vi "S4GUI.vi"() -> ()   [LabVIEW 2018] (continued)
                n1359 = call-dynamic "Read Interface.vi"("error in (no error)"=w3056, "Channel in"=w3057) -> ("error out"=w3047:errorcluster, "Interface.lvclass"=w3046:refnum<class "Interface.lvclass">, "Channel out"=w3059:refnum<class "Channel.lvclass">)  [unwired: 7 in]
                n1360 = call-dynamic "Get CCD_Config.vi"("error in (no error)"=w3047, "Interface in"=w3046) -> ("error out"=w3049:errorcluster, "output cluster"=w3050:T24, "Interface out"=w3045:refnum<class "Interface.lvclass">)  [unwired: 7 in]
                n1361 = Bundle By Name(cluster=w3050, "TRIGGER_MODE"=w3023) -> (w3048:T24)
                n1362 = call-dynamic "Set CCD_Config.vi"("error in (no error)"=w3049, "input cluster"=w3048, "Interface in"=w3045) -> ("error out"=w3051:errorcluster, "Interface out"=w3044:refnum<class "Interface.lvclass">)  [unwired: 7 in]
                n1363 = Flatten To String(anything=w3048, error in (no error)=w3051) -> (data string=w3053:string, error out=w3052:errorcluster)  [unwired: 2 in, 1 out]
                n1364 = call "Write flatted cluster.vi"("error in (no error)"=w3052, "flatted cluster"=w3053, "Interface in"=w3044) -> ("error out"=w3042:errorcluster, "Interface out"=w3043:refnum<class "Interface.lvclass">)  [unwired: 7 in]
                n1365 = call-dynamic "Write Interface.vi"("error in (no error)"=w3042, "Interface.lvclass"=w3043, "Channel in"=w3059) -> ("error out"=w3037:errorcluster, "Channel out"=w3036:refnum<class "Channel.lvclass">)  [unwired: 7 in]
                n1366 = call "Write section_name.vi"("error in (no error)"=w3037, "section_name"="CCD_ACS1", "Channel in"=w3036) -> ("error out"=w3038:errorcluster, "Channel out"=w3033:refnum<class "Channel.lvclass">)  [unwired: 7 in]
                n1367 = call-dynamic "save config.vi"("error in (no error)"=w3038, "file config"="lastsaved.cfg", "Channel in"=w3033) -> ("error out"=w3026:errorcluster, "Channel out"=w3027:refnum<class "Channel.lvclass">)  [unwired: 7 in]
                n1368 = call-dynamic "Read State Machine.vi"("error in (no error)"=w3026, "Device in"=w3027) -> ("error out"=w3041:errorcluster, "State Machine.lvclass"=w3031:refnum<class "State Machine.lvclass">, "Device out"=w3032:refnum<class "Channel.lvclass">)  [unwired: 7 in]
                n1369 = call-dynamic "Write State.vi"("error in (no error)"=w3041, "State"=60, "State Machine in"=w3031) -> ("error out"=w3040:errorcluster, "State Machine out"=w3030:refnum<class "State Machine.lvclass">)  [unwired: 7 in]
                n1370 = call-dynamic "Write State Machine.vi"("error in (no error)"=w3040, "State Machine.lvclass"=w3030, "Device in"=w3032) -> ("error out"=w3028:errorcluster, "Device out"=w3029:refnum<class "Channel.lvclass">)  [unwired: 7 in]
                n1371 = call-dynamic "Write Channel.vi"("error in (no error)"=w3028, "Channel.lvclass"=w3029, "Acquisition in"=w3058) -> ("error out"=w3055:errorcluster, "Acquisition out"=w3054:refnum<class "Acquisition.lvclass">)  [unwired: 7 in]
              }
            }
            n1372 = call-dynamic "Write AcquisitionA.vi"("error in (no error)"=w2860, "Acquisition.lvclass"=w2861, "S4ACS_GUI in"=w2862) -> ("error out"=w2868:errorcluster, "S4ACS_GUI out"=w2871:refnum<class "S4GUI.lvclass">)  [unwired: 7 in]
            n1373 = call "Write AcquisitionB.vi"("error in (no error)"=w2858, "Acquisition.lvclass"=w2859, "S4ACS_GUI in"=w2871) -> ("error out"=w2867:errorcluster, "S4ACS_GUI out"=w2870:refnum<class "S4GUI.lvclass">)  [unwired: 7 in]
            n1374 = call-dynamic "Write AcquisitionC.vi"("error in (no error)"=w2856, "Acquisition.lvclass"=w2857, "S4ACS_GUI in"=w2870) -> ("error out"=w2866:errorcluster, "S4ACS_GUI out"=w2869:refnum<class "S4GUI.lvclass">)  [unwired: 7 in]
            n1375 = call-dynamic "Write AcquisitionD.vi"("error in (no error)"=w2854, "Acquisition.lvclass"=w2855, "S4ACS_GUI in"=w2869) -> ("error out"=w2865:errorcluster, "S4ACS_GUI out"=w2864:refnum<class "S4GUI.lvclass">)  [unwired: 7 in]
            n1376 = Merge Errors(w2868, w2867, w2866, w2865) -> (w2863:errorcluster)
          }
        }
        n1377 = call-dynamic "Write sync.vi"("error in (no error)"=w2602, "sync"=w2628, "S4ACS_GUI in"=w2603) -> ("error out"=w2627:errorcluster, "S4ACS_GUI out"=w2604:refnum<class "S4GUI.lvclass">)  [unwired: 7 in]
        n1378 = property on="#Cycles Done" class="Slide (strict)"(error in=w2627, "DisabledEnum"=w2625) -> (error out=w2626:errorcluster)  [unwired: 1 in, 1 out]
        n1379 = property on="Cycles Done ch1" class="Slide (strict)"(error in=w2626, "DisabledEnum"=w2605) -> (error out=w2624:errorcluster)  [unwired: 1 in, 1 out]
        n1380 = property on="Cycles Done ch2" class="Slide (strict)"(error in=w2624, "DisabledEnum"=w2605) -> (error out=w2608:errorcluster)  [unwired: 1 in, 1 out]
        n1381 = property on="Cycles Done ch3" class="Slide (strict)"(error in=w2608, "DisabledEnum"=w2605) -> (error out=w2607:errorcluster)  [unwired: 1 in, 1 out]
        n1382 = property on="Cycles Done ch4" class="Slide (strict)"(error in=w2607, "DisabledEnum"=w2605) -> (error out=w2606:errorcluster)  [unwired: 1 in, 1 out]
        n1383 = property on="Stop SM" class="Bool"(error in=w2606, "DisabledEnum"=w2630) -> (error out=w2632:errorcluster)  [unwired: 1 in, 1 out]
        n1384 = property on="Start SM" class="Bool"(error in=w2632, "DisabledEnum"=w2630) -> (error out=w2631:errorcluster)  [unwired: 1 in, 1 out]
        n1385 = property on="Abort SM" class="Bool"(error in=w2631, "DisabledEnum"=w2630) -> (error out=w2629:errorcluster)  [unwired: 1 in, 1 out]
        n1386 = property on="Start ch1" class="Bool"(error in=w2629, "DisabledEnum"=w2611, "BoolText.Text"=w2622) -> (error out=w2623:errorcluster)  [unwired: 1 in, 1 out]
        n1387 = property on="Start ch2" class="Bool"(error in=w2623, "DisabledEnum"=w2611, "BoolText.Text"=w2622) -> (error out=w2614:errorcluster)  [unwired: 1 in, 1 out]
        n1388 = property on="Pause ch1" class="Bool"(error in=w2614, "DisabledEnum"=w2611, "BoolText.Text"=w2617) -> (error out=w2621:errorcluster)  [unwired: 1 in, 1 out]
        n1389 = property on="Pause ch2" class="Bool"(error in=w2621, "DisabledEnum"=w2611, "BoolText.Text"=w2617) -> (error out=w2613:errorcluster)  [unwired: 1 in, 1 out]
        n1390 = property on="Stop ch1" class="Bool"(error in=w2613, "DisabledEnum"=w2611, "BoolText.Text"=w2615) -> (error out=w2620:errorcluster)  [unwired: 1 in, 1 out]
        n1391 = property on="Stop ch2" class="Bool"(error in=w2620, "DisabledEnum"=w2611, "BoolText.Text"=w2615) -> (error out=w2609:errorcluster)  [unwired: 1 in, 1 out]
        n1392 = property on="Abort ch1" class="Bool"(error in=w2609, "DisabledEnum"=w2611, "BoolText.Text"=w2610) -> (error out=w2619:errorcluster)  [unwired: 1 in, 1 out]
        n1393 = property on="Abort ch2" class="Bool"(error in=w2619, "DisabledEnum"=w2611, "BoolText.Text"=w2610) -> (error out=w2601:errorcluster)  [unwired: 1 in, 1 out]
        n1394 = property on="Pause ch3" class="Bool"(error in=w2601, "DisabledEnum"=w2611, "BoolText.Text"=w2617) -> (error out=w2618:errorcluster)  [unwired: 1 in, 1 out]
        n1395 = property on="Pause ch4" class="Bool"(error in=w2618, "DisabledEnum"=w2611, "BoolText.Text"=w2617) -> (error out=w2598:errorcluster)  [unwired: 1 in, 1 out]
        n1396 = property on="Stop ch3" class="Bool"(error in=w2598, "DisabledEnum"=w2611, "BoolText.Text"=w2615) -> (error out=w2616:errorcluster)  [unwired: 1 in, 1 out]
        n1397 = property on="Stop ch4" class="Bool"(error in=w2616, "DisabledEnum"=w2611, "BoolText.Text"=w2615) -> (error out=w2599:errorcluster)  [unwired: 1 in, 1 out]
        n1398 = property on="Abort ch3" class="Bool"(error in=w2599, "DisabledEnum"=w2611, "BoolText.Text"=w2610) -> (error out=w2612:errorcluster)  [unwired: 1 in, 1 out]
        n1399 = property on="Abort ch4" class="Bool"(error in=w2612, "DisabledEnum"=w2611, "BoolText.Text"=w2610) -> (error out=w2600:errorcluster)  [unwired: 1 in, 1 out]
      }
      event "ExtSync": Value Change {
        n1400 = event-data() -> ("NewVal"=w3143:bool)  [unwired: 1 in]
        n1401 = Not(x=w3143) -> (.not. x?=w3062:bool)
        n1402 = call-dynamic "Read Sync Box.lvclass.vi"("error in (no error)"=w3146, "SPARC4_AC in"=w3155) -> ("error out"=w3148:errorcluster, "Sync Box.lvclass"=w3154:refnum<class "Sync Box.lvclass">, "SPARC4_AC out"=w3151:refnum<class "S4GUI.lvclass">)  [unwired: 7 in]
        n1403 = call-dynamic "Read Stream.vi"("error in (no error)"=w3148, "Server in"=w3154) -> ("error out"=w3147:errorcluster, "Stream.lvclass"=w3156:refnum<class "Stream.lvclass">, "Server out"=w3145:refnum<class "Sync Box.lvclass">)  [unwired: 7 in]
        n1404 = case shown="True" w3143 {
          tunnel: [w3161 w3178] -> w3149
          tunnel: w3156 -> [w3163 w3166]
          tunnel: [w3162 w3174] -> w3153
          tunnel: w3147 -> [w3159 w3165]
          tunnel: w3145 -> [w3160 w3168]
          tunnel: [w3157 w3167] -> w3144
          frame False {
            n1405 = call-dynamic "ReleaseQueueTCPIP.vi"("error in (no error)"=w3159, "Server in"=w3160) -> ("error out"=w3158:errorcluster, "Server out"=w3157:refnum<class "Sync Box.lvclass">)  [unwired: 8 in]
            n1406 = call-dynamic "End.vi"("error in (no error)"=w3158, "Stream in"=w3163) -> ("error out"=w3161:errorcluster, "Stream out"=w3162:refnum<class "Stream.lvclass">)  [unwired: 8 in]
          }
          frame True {
            w3171 = errorcluster {"status"=FALSE, "code"=0, "source"=""} ("error in (no error)")
            w3190 = FALSE ("Wait Until Done")
            w3185 = FALSE ("Wait Until Done")
            n1407 = call-dynamic "Send TCP Param.vi"("error in (no error)"=w3165, "Server in"=w3168) -> ("error out"=w3164:errorcluster, "Server out"=w3167:refnum<class "Sync Box.lvclass">)  [unwired: 8 in]
            n1408 = call-dynamic "Read StreamRX filename.vi"("error in (no error)"=w3164, "Stream in"=w3166) -> ("error out"=w3181:errorcluster, "StreamRX filename"=w3182:string, "Stream out"=w3177:refnum<class "Stream.lvclass">)  [unwired: 7 in]
            n1409 = call <vilib>:"Application Directory.vi"() -> ("Application Directory"=w3187:path)
            n1410 = call <vilib>:"Application Directory.vi"() -> ("Application Directory"=w3191:path)
            n1411 = Build Path(base path=w3191, name or relative path=w3182) -> (appended path=w3192:path)
            n1412 = Open VI Reference(vi path=w3192, error in (no error)=w3181) -> (vi reference=w3184:refnum<vi>, error out=w3183:errorcluster)  [unwired: 4 in]
            n1413 = invoke class="VI" method="Run VI"(reference=w3184, error in=w3183, "Wait until done"=w3185, "Auto Dispose Ref"=w3185) -> (reference out=w3173:refnum<vi>, error out=→"error out 7":errorcluster)  [unwired: 1 in, 3 out]
            n1414 = call-dynamic "Write stream writer vi ref.vi"("error in (no error)"=w3171, "stream writer vi ref"=w3173, "Stream in"=w3177) -> ("error out"=w3179:errorcluster, "Stream out"=w3176:refnum<class "Stream.lvclass">)  [unwired: 7 in]
            n1415 = call-dynamic "Read StreamTX filename.vi"("Stream in"=w3176) -> ("StreamTX filename"=w3180:string, "Stream out"=w3175:refnum<class "Stream.lvclass">)  [unwired: 8 in, 1 out]
            n1416 = Build Path(base path=w3187, name or relative path=w3180) -> (appended path=w3186:path)
            n1417 = Open VI Reference(vi path=w3186, error in (no error)=w3179) -> (vi reference=w3188:refnum<vi>, error out=w3189:errorcluster)  [unwired: 4 in]
            n1418 = invoke class="VI" method="Run VI"(reference=w3188, error in=w3189, "Wait until done"=w3190, "Auto Dispose Ref"=w3190) -> (reference out=w3172:refnum<vi>, error out=→"error out 8":errorcluster)  [unwired: 1 in, 3 out]
            n1419 = call-dynamic "Write stream reader vi ref.vi"("error in (no error)"=w3171, "stream reader vi ref"=w3172, "Stream in"=w3175) -> ("error out"=w3178:errorcluster, "Stream out"=w3174:refnum<class "Stream.lvclass">)  [unwired: 7 in]
          }
        }
        n1420 = call-dynamic "Write Stream.vi"("error in (no error)"=w3149, "Stream.lvclass"=w3153, "Server in"=w3144) -> ("error out"=w3150:errorcluster, "Server out"=w3152:refnum<class "Sync Box.lvclass">)  [unwired: 7 in]
        n1421 = call-dynamic "Write Sync Box.lvclass.vi"("error in (no error)"=w3150, "Sync Box.lvclass"=w3152, "SPARC4_AC in"=w3151) -> ("error out"=w3141:errorcluster, "SPARC4_AC out"=w3142:refnum<class "S4GUI.lvclass">)  [unwired: 7 in]
        n1422 = call-dynamic "Read AcquisitionC.vi"("error in (no error)"=w3141, "S4ACS_GUI in"=w3142) -> ("error out"=w3084:errorcluster, "Acquisition.lvclass"=w3085:refnum<class "Acquisition.lvclass">)  [unwired: 7 in, 1 out]
        n1423 = call-dynamic "Read AcquisitionA.vi"("error in (no error)"=w3141, "S4ACS_GUI in"=w3142) -> ("error out"=w3121:errorcluster, "Acquisition.lvclass"=w3120:refnum<class "Acquisition.lvclass">, "S4ACS_GUI out"=w3137:refnum<class "S4GUI.lvclass">)  [unwired: 7 in]
        n1424 = call "Read AcquisitionB.vi"("error in (no error)"=w3141, "S4ACS_GUI in"=w3142) -> ("error out"=w3101:errorcluster, "Acquisition.lvclass"=w3102:refnum<class "Acquisition.lvclass">)  [unwired: 7 in, 1 out]
        n1425 = call-dynamic "Read AcquisitionD.vi"("error in (no error)"=w3141, "S4ACS_GUI in"=w3142) -> ("error out"=w3067:errorcluster, "Acquisition.lvclass"=w3068:refnum<class "Acquisition.lvclass">)  [unwired: 7 in, 1 out]
        n1426 = call-dynamic "Read Channel.vi"("error in (no error)"=w3067, "Acquisition in"=w3068) -> ("error out"=w3070:errorcluster, "Channel.lvclass"=w3072:refnum<class "Channel.lvclass">, "Acquisition out"=w3081:refnum<class "Acquisition.lvclass">)  [unwired: 7 in]
        n1427 = call-dynamic "Read Channel.vi"("error in (no error)"=w3084, "Acquisition in"=w3085) -> ("error out"=w3087:errorcluster, "Channel.lvclass"=w3089:refnum<class "Channel.lvclass">, "Acquisition out"=w3098:refnum<class "Acquisition.lvclass">)  [unwired: 7 in]
        n1428 = call-dynamic "Read Channel.vi"("error in (no error)"=w3101, "Acquisition in"=w3102) -> ("error out"=w3104:errorcluster, "Channel.lvclass"=w3106:refnum<class "Channel.lvclass">, "Acquisition out"=w3115:refnum<class "Acquisition.lvclass">)  [unwired: 7 in]
        n1429 = call-dynamic "Read Channel.vi"("error in (no error)"=w3121, "Acquisition in"=w3120) -> ("error out"=w3117:errorcluster, "Channel.lvclass"=w3119:refnum<class "Channel.lvclass">, "Acquisition out"=w3130:refnum<class "Acquisition.lvclass">)  [unwired: 7 in]
        n1430 = call-dynamic "Write wait_expose.vi"("error in (no error)"=w3070, "wait_expose"=w3062, "Channel in"=w3072) -> ("error out"=w3069:errorcluster, "Channel out"=w3071:refnum<class "Channel.lvclass">)  [unwired: 7 in]
        n1431 = call-dynamic "Write wait_expose.vi"("error in (no error)"=w3087, "wait_expose"=w3062, "Channel in"=w3089) -> ("error out"=w3086:errorcluster, "Channel out"=w3088:refnum<class "Channel.lvclass">)  [unwired: 7 in]
        n1432 = call-dynamic "Write wait_expose.vi"("error in (no error)"=w3104, "wait_expose"=w3062, "Channel in"=w3106) -> ("error out"=w3103:errorcluster, "Channel out"=w3105:refnum<class "Channel.lvclass">)  [unwired: 7 in]
        n1433 = call-dynamic "Write wait_expose.vi"("error in (no error)"=w3117, "wait_expose"=w3062, "Channel in"=w3119) -> ("error out"=w3116:errorcluster, "Channel out"=w3118:refnum<class "Channel.lvclass">)  [unwired: 7 in]
        n1434 = call-dynamic "Read State Machine.vi"("error in (no error)"=w3069, "Device in"=w3071) -> ("error out"=w3080:errorcluster, "State Machine.lvclass"=w3076:refnum<class "State Machine.lvclass">, "Device out"=w3077:refnum<class "Channel.lvclass">)  [unwired: 7 in]
        n1435 = call-dynamic "Read State Machine.vi"("error in (no error)"=w3086, "Device in"=w3088) -> ("error out"=w3097:errorcluster, "State Machine.lvclass"=w3093:refnum<class "State Machine.lvclass">, "Device out"=w3094:refnum<class "Channel.lvclass">)  [unwired: 7 in]
        n1436 = call-dynamic "Read State Machine.vi"("error in (no error)"=w3103, "Device in"=w3105) -> ("error out"=w3114:errorcluster, "State Machine.lvclass"=w3110:refnum<class "State Machine.lvclass">, "Device out"=w3111:refnum<class "Channel.lvclass">)  [unwired: 7 in]
        n1437 = call-dynamic "Read State Machine.vi"("error in (no error)"=w3116, "Device in"=w3118) -> ("error out"=w3129:errorcluster, "State Machine.lvclass"=w3125:refnum<class "State Machine.lvclass">, "Device out"=w3126:refnum<class "Channel.lvclass">)  [unwired: 7 in]
        n1438 = call-dynamic "Write State.vi"("error in (no error)"=w3080, "State"=40, "State Machine in"=w3076) -> ("error out"=w3079:errorcluster, "State Machine out"=w3075:refnum<class "State Machine.lvclass">)  [unwired: 7 in]
        n1439 = call-dynamic "Write State.vi"("error in (no error)"=w3097, "State"=40, "State Machine in"=w3093) -> ("error out"=w3096:errorcluster, "State Machine out"=w3092:refnum<class "State Machine.lvclass">)  [unwired: 7 in]
        n1440 = call-dynamic "Write State.vi"("error in (no error)"=w3114, "State"=40, "State Machine in"=w3110) -> ("error out"=w3113:errorcluster, "State Machine out"=w3109:refnum<class "State Machine.lvclass">)  [unwired: 7 in]
        n1441 = call-dynamic "Write State.vi"("error in (no error)"=w3129, "State"=40, "State Machine in"=w3125) -> ("error out"=w3128:errorcluster, "State Machine out"=w3124:refnum<class "State Machine.lvclass">)  [unwired: 7 in]
        n1442 = call-dynamic "Write State Machine.vi"("error in (no error)"=w3079, "State Machine.lvclass"=w3075, "Device in"=w3077) -> ("error out"=w3073:errorcluster, "Device out"=w3074:refnum<class "Channel.lvclass">)  [unwired: 7 in]
        n1443 = call-dynamic "Write State Machine.vi"("error in (no error)"=w3096, "State Machine.lvclass"=w3092, "Device in"=w3094) -> ("error out"=w3090:errorcluster, "Device out"=w3091:refnum<class "Channel.lvclass">)  [unwired: 7 in]
        n1444 = call-dynamic "Write State Machine.vi"("error in (no error)"=w3113, "State Machine.lvclass"=w3109, "Device in"=w3111) -> ("error out"=w3107:errorcluster, "Device out"=w3108:refnum<class "Channel.lvclass">)  [unwired: 7 in]
        n1445 = call-dynamic "Write State Machine.vi"("error in (no error)"=w3128, "State Machine.lvclass"=w3124, "Device in"=w3126) -> ("error out"=w3122:errorcluster, "Device out"=w3123:refnum<class "Channel.lvclass">)  [unwired: 7 in]
        n1446 = call-dynamic "Write Channel.vi"("error in (no error)"=w3073, "Channel.lvclass"=w3074, "Acquisition in"=w3081) -> ("error out"=w3065:errorcluster, "Acquisition out"=w3066:refnum<class "Acquisition.lvclass">)  [unwired: 7 in]
        n1447 = call-dynamic "Write Channel.vi"("error in (no error)"=w3090, "Channel.lvclass"=w3091, "Acquisition in"=w3098) -> ("error out"=w3083:errorcluster, "Acquisition out"=w3082:refnum<class "Acquisition.lvclass">)  [unwired: 7 in]
        n1448 = call-dynamic "Write Channel.vi"("error in (no error)"=w3107, "Channel.lvclass"=w3108, "Acquisition in"=w3115) -> ("error out"=w3100:errorcluster, "Acquisition out"=w3099:refnum<class "Acquisition.lvclass">)  [unwired: 7 in]
        n1449 = call-dynamic "Write Channel.vi"("error in (no error)"=w3122, "Channel.lvclass"=w3123, "Acquisition in"=w3130) -> ("error out"=w3135:errorcluster, "Acquisition out"=w3136:refnum<class "Acquisition.lvclass">)  [unwired: 7 in]
        n1450 = call-dynamic "Write AcquisitionA.vi"("error in (no error)"=w3135, "Acquisition.lvclass"=w3136, "S4ACS_GUI in"=w3137) -> ("error out"=w3134:errorcluster, "S4ACS_GUI out"=w3140:refnum<class "S4GUI.lvclass">)  [unwired: 7 in]
        n1451 = call "Write AcquisitionB.vi"("error in (no error)"=w3100, "Acquisition.lvclass"=w3099, "S4ACS_GUI in"=w3140) -> ("error out"=w3133:errorcluster, "S4ACS_GUI out"=w3139:refnum<class "S4GUI.lvclass">)  [unwired: 7 in]
        n1452 = call-dynamic "Write AcquisitionC.vi"("error in (no error)"=w3083, "Acquisition.lvclass"=w3082, "S4ACS_GUI in"=w3139) -> ("error out"=w3132:errorcluster, "S4ACS_GUI out"=w3138:refnum<class "S4GUI.lvclass">)  [unwired: 7 in]
        n1453 = call-dynamic "Write AcquisitionD.vi"("error in (no error)"=w3065, "Acquisition.lvclass"=w3066, "S4ACS_GUI in"=w3138) -> ("error out"=w3131:errorcluster, "S4ACS_GUI out"=w3064:refnum<class "S4GUI.lvclass">)  [unwired: 7 in]
        n1454 = Merge Errors(w3134, w3133, w3132, w3131) -> (w3063:errorcluster)
        n1455 = call-dynamic "Write mode EXPOSE.vi"("error in (no error)"=w3063, "mode EXPOSE"=w3062, "S4GUI in"=w3064) -> ("error out"=w3060:errorcluster, "S4GUI out"=w3061:refnum<class "S4GUI.lvclass">)  [unwired: 7 in]
      }
      event "Start SM": Value Change {
        n1456 = event-data() -> ()  [unwired: 1 in, 6 out]
        n1457 = call-dynamic "Read Obs_state.vi"("error in (no error)"=w3212, "S4ACS_GUI in"=w3213) -> ("error out"=w3197:errorcluster, "Obs_state"=w3210:u32, "S4ACS_GUI out"=w3199:refnum<class "S4GUI.lvclass">)  [unwired: 7 in]
        n1458 = call "Read Instrument.lvclass.vi"("error in (no error)"=w3197, "S4ACS_GUI in"=w3199) -> ("error out"=w3195:errorcluster, "Instrument.lvclass"=w3196:refnum<class "Instrument.lvclass">, "S4ACS_GUI out"=w3198:refnum<class "S4GUI.lvclass">)  [unwired: 7 in]
        n1459 = Not Equal?(x=w3210, y=u32 400) -> (x != y?=w3209:bool)
        n1460 = call-dynamic "Read mode.vi"("error in (no error)"=w3195, "Instrument in"=w3196) -> ("error out"=w3194:errorcluster, "mode"=w3193:bool)  [unwired: 7 in, 1 out]
        n1461 = case shown="True" w3209 {
          tunnel: w3198 -> [w3280 w3333]
          tunnel: w3194 -> [w3276 w3331]
          tunnel: [w3215 w3346] -> w3203
          tunnel: [w3214 w3344] -> w3207
          tunnel: w3205 -> [_ w3353]
          tunnel: w3204 -> [_ w3352]
          tunnel: w3202 -> [_ w3351]
          tunnel: w3201 -> [_ w3350]
          tunnel: w3200 -> [_ w3349]
          tunnel: w3193 -> [_ w3348]
          frame False {
            # "Obs_state=400 (PAUSED), então retoma a execução do estado onde parou."
            n1462 = call-dynamic "Read Obs_prevstate.vi"("error in (no error)"=w3276, "S4ACS_GUI in"=w3280) -> ("error out"=w3277:errorcluster, "Obs_prevstate"=w3279:u32, "S4ACS_GUI out"=w3278:refnum<class "S4GUI.lvclass">)  [unwired: 7 in]
            n1463 = call-dynamic "Write Obs_state.vi"("error in (no error)"=w3277, "Obs_state"=w3279, "S4ACS_GUI in"=w3278) -> ("error out"=w3216:errorcluster, "S4ACS_GUI out"=w3217:refnum<class "S4GUI.lvclass">)  [unwired: 7 in]
            n1464 = call-dynamic "Read AcquisitionA.vi"("error in (no error)"=w3216, "S4ACS_GUI in"=w3217) -> ("error out"=w3270:errorcluster, "Acquisition.lvclass"=w3274:refnum<class "Acquisition.lvclass">, "S4ACS_GUI out"=w3275:refnum<class "S4GUI.lvclass">)  [unwired: 7 in]
            n1465 = call-dynamic "Read Channel.vi"("error in (no error)"=w3270, "Acquisition in"=w3274) -> ("error out"=w3241:errorcluster, "Channel.lvclass"=w3242:refnum<class "Channel.lvclass">, "Acquisition out"=w3273:refnum<class "Acquisition.lvclass">)  [unwired: 7 in]
            n1466 = call "Read connected.vi"("error in (no error)"=w3241, "Device in"=w3242) -> ("error out"=w3240:errorcluster, "connected"=w3239:bool, "Device out"=w3243:refnum<class "Channel.lvclass">)  [unwired: 7 in]
            n1467 = case shown="True" w3239 {
              tunnel: w3243 -> [w3318 w3328]
              tunnel: [w3318 w3326] -> w3271
              tunnel: w3240 -> [w3317 w3323]
              tunnel: [w3317 w3321] -> w3269
              frame False {
              }
              frame True {
                n1468 = call-dynamic "Read State Machine.vi"("error in (no error)"=w3323, "Device in"=w3328) -> ("error out"=w3319:errorcluster, "State Machine.lvclass"=w3320:refnum<class "State Machine.lvclass">, "Device out"=w3327:refnum<class "Channel.lvclass">)  [unwired: 7 in]
                n1469 = call "Next State.vi"("error in (no error)"=w3319, "New_State"=96, "State Machine in"=w3320) -> ("error out"=w3322:errorcluster, "State Machine out"=w3325:refnum<class "State Machine.lvclass">)  [unwired: 7 in]
                n1470 = call-dynamic "Write State Machine.vi"("error in (no error)"=w3322, "State Machine.lvclass"=w3325, "Device in"=w3327) -> ("error out"=w3321:errorcluster, "Device out"=w3326:refnum<class "Channel.lvclass">)  [unwired: 7 in]
              }
            }
            n1471 = call-dynamic "Write Channel.vi"("error in (no error)"=w3269, "Channel.lvclass"=w3271, "Acquisition in"=w3273) -> ("error out"=w3268:errorcluster, "Acquisition out"=w3272:refnum<class "Acquisition.lvclass">)  [unwired: 7 in]
            n1472 = call-dynamic "Write AcquisitionA.vi"("error in (no error)"=w3268, "Acquisition.lvclass"=w3272, "S4ACS_GUI in"=w3275) -> ("error out"=w3249:errorcluster, "S4ACS_GUI out"=w3246:refnum<class "S4GUI.lvclass">)  [unwired: 7 in]
            n1473 = call "Read AcquisitionB.vi"("error in (no error)"=w3249, "S4ACS_GUI in"=w3246) -> ("error out"=w3263:errorcluster, "Acquisition.lvclass"=w3266:refnum<class "Acquisition.lvclass">, "S4ACS_GUI out"=w3267:refnum<class "S4GUI.lvclass">)  [unwired: 7 in]
            n1474 = call-dynamic "Read Channel.vi"("error in (no error)"=w3263, "Acquisition in"=w3266) -> ("error out"=w3234:errorcluster, "Channel.lvclass"=w3235:refnum<class "Channel.lvclass">, "Acquisition out"=w3265:refnum<class "Acquisition.lvclass">)  [unwired: 7 in]
            n1475 = call "Read connected.vi"("error in (no error)"=w3234, "Device in"=w3235) -> ("error out"=w3237:errorcluster, "connected"=w3236:bool, "Device out"=w3238:refnum<class "Channel.lvclass">)  [unwired: 7 in]
            n1476 = case shown="True" w3236 {
              tunnel: w3238 -> [w3306 w3316]
              tunnel: [w3306 w3314] -> w3232
              tunnel: w3237 -> [w3305 w3311]
              tunnel: [w3305 w3309] -> w3233
              frame False {
              }
              frame True {
                n1477 = call-dynamic "Read State Machine.vi"("error in (no error)"=w3311, "Device in"=w3316) -> ("error out"=w3307:errorcluster, "State Machine.lvclass"=w3308:refnum<class "State Machine.lvclass">, "Device out"=w3315:refnum<class "Channel.lvclass">)  [unwired: 7 in]
                n1478 = call "Next State.vi"("error in (no error)"=w3307, "New_State"=96, "State Machine in"=w3308) -> ("error out"=w3310:errorcluster, "State Machine out"=w3313:refnum<class "State Machine.lvclass">)  [unwired: 7 in]
                n1479 = call-dynamic "Write State Machine.vi"("error in (no error)"=w3310, "State Machine.lvclass"=w3313, "Device in"=w3315) -> ("error out"=w3309:errorcluster, "Device out"=w3314:refnum<class "Channel.lvclass">)  [unwired: 7 in]
              }
            }
            n1480 = call-dynamic "Write Channel.vi"("error in (no error)"=w3233, "Channel.lvclass"=w3232, "Acquisition in"=w3265) -> ("error out"=w3262:errorcluster, "Acquisition out"=w3264:refnum<class "Acquisition.lvclass">)  [unwired: 7 in]
            n1481 = call "Write AcquisitionB.vi"("error in (no error)"=w3262, "Acquisition.lvclass"=w3264, "S4ACS_GUI in"=w3267) -> ("error out"=w3248:errorcluster, "S4ACS_GUI out"=w3245:refnum<class "S4GUI.lvclass">)  [unwired: 7 in]
            n1482 = call-dynamic "Read AcquisitionC.vi"("error in (no error)"=w3248, "S4ACS_GUI in"=w3245) -> ("error out"=w3257:errorcluster, "Acquisition.lvclass"=w3260:refnum<class "Acquisition.lvclass">, "S4ACS_GUI out"=w3261:refnum<class "S4GUI.lvclass">)  [unwired: 7 in]
            n1483 = call-dynamic "Read Channel.vi"("error in (no error)"=w3257, "Acquisition in"=w3260) -> ("error out"=w3227:errorcluster, "Channel.lvclass"=w3228:refnum<class "Channel.lvclass">, "Acquisition out"=w3259:refnum<class "Acquisition.lvclass">)  [unwired: 7 in]
            n1484 = call "Read connected.vi"("error in (no error)"=w3227, "Device in"=w3228) -> ("error out"=w3230:errorcluster, "connected"=w3229:bool, "Device out"=w3231:refnum<class "Channel.lvclass">)  [unwired: 7 in]
            n1485 = case shown="True" w3229 {
              tunnel: w3231 -> [w3294 w3304]
              tunnel: [w3294 w3302] -> w3226
              tunnel: w3230 -> [w3293 w3299]
              tunnel: [w3293 w3297] -> w3225
              frame False {
              }
              frame True {
                n1486 = call-dynamic "Read State Machine.vi"("error in (no error)"=w3299, "Device in"=w3304) -> ("error out"=w3295:errorcluster, "State Machine.lvclass"=w3296:refnum<class "State Machine.lvclass">, "Device out"=w3303:refnum<class "Channel.lvclass">)  [unwired: 7 in]
                n1487 = call "Next State.vi"("error in (no error)"=w3295, "New_State"=96, "State Machine in"=w3296) -> ("error out"=w3298:errorcluster, "State Machine out"=w3301:refnum<class "State Machine.lvclass">)  [unwired: 7 in]
                n1488 = call-dynamic "Write State Machine.vi"("error in (no error)"=w3298, "State Machine.lvclass"=w3301, "Device in"=w3303) -> ("error out"=w3297:errorcluster, "Device out"=w3302:refnum<class "Channel.lvclass">)  [unwired: 7 in]
              }
            }
            n1489 = call-dynamic "Write Channel.vi"("error in (no error)"=w3225, "Channel.lvclass"=w3226, "Acquisition in"=w3259) -> ("error out"=w3256:errorcluster, "Acquisition out"=w3258:refnum<class "Acquisition.lvclass">)  [unwired: 7 in]
            n1490 = call-dynamic "Write AcquisitionC.vi"("error in (no error)"=w3256, "Acquisition.lvclass"=w3258, "S4ACS_GUI in"=w3261) -> ("error out"=w3247:errorcluster, "S4ACS_GUI out"=w3244:refnum<class "S4GUI.lvclass">)  [unwired: 7 in]
            n1491 = call-dynamic "Read AcquisitionD.vi"("error in (no error)"=w3247, "S4ACS_GUI in"=w3244) -> ("error out"=w3251:errorcluster, "Acquisition.lvclass"=w3254:refnum<class "Acquisition.lvclass">, "S4ACS_GUI out"=w3255:refnum<class "S4GUI.lvclass">)  [unwired: 7 in]
            n1492 = call-dynamic "Read Channel.vi"("error in (no error)"=w3251, "Acquisition in"=w3254) -> ("error out"=w3220:errorcluster, "Channel.lvclass"=w3221:refnum<class "Channel.lvclass">, "Acquisition out"=w3253:refnum<class "Acquisition.lvclass">)  [unwired: 7 in]
            n1493 = call "Read connected.vi"("error in (no error)"=w3220, "Device in"=w3221) -> ("error out"=w3223:errorcluster, "connected"=w3222:bool, "Device out"=w3224:refnum<class "Channel.lvclass">)  [unwired: 7 in]
            n1494 = case shown="True" w3222 {
              tunnel: w3224 -> [w3282 w3292]
              tunnel: [w3282 w3290] -> w3219
              tunnel: w3223 -> [w3281 w3287]
              tunnel: [w3281 w3285] -> w3218
              frame False {
              }
              frame True {
                n1495 = call-dynamic "Read State Machine.vi"("error in (no error)"=w3287, "Device in"=w3292) -> ("error out"=w3283:errorcluster, "State Machine.lvclass"=w3284:refnum<class "State Machine.lvclass">, "Device out"=w3291:refnum<class "Channel.lvclass">)  [unwired: 7 in]
                n1496 = call "Next State.vi"("error in (no error)"=w3283, "New_State"=96, "State Machine in"=w3284) -> ("error out"=w3286:errorcluster, "State Machine out"=w3289:refnum<class "State Machine.lvclass">)  [unwired: 7 in]
                n1497 = call-dynamic "Write State Machine.vi"("error in (no error)"=w3286, "State Machine.lvclass"=w3289, "Device in"=w3291) -> ("error out"=w3285:errorcluster, "Device out"=w3290:refnum<class "Channel.lvclass">)  [unwired: 7 in]
              }
            }
            n1498 = call-dynamic "Write Channel.vi"("error in (no error)"=w3218, "Channel.lvclass"=w3219, "Acquisition in"=w3253) -> ("error out"=w3250:errorcluster, "Acquisition out"=w3252:refnum<class "Acquisition.lvclass">)  [unwired: 7 in]
            n1499 = call-dynamic "Write AcquisitionD.vi"("error in (no error)"=w3250, "Acquisition.lvclass"=w3252, "S4ACS_GUI in"=w3255) -> ("error out"=w3214:errorcluster, "S4ACS_GUI out"=w3215:refnum<class "S4GUI.lvclass">)  [unwired: 7 in]
          }
          frame True {
            n1500 = call "Read Instrument.lvclass.vi"("error in (no error)"=w3331, "S4ACS_GUI in"=w3333) -> ("error out"=w3335:errorcluster, "Instrument.lvclass"=w3337:refnum<class "Instrument.lvclass">, "S4ACS_GUI out"=w3332:refnum<class "S4GUI.lvclass">)  [unwired: 7 in]
            n1501 = call "Read WPROT.vi"("error in (no error)"=w3335, "Instrument in"=w3337) -> ("error out"=w3334:errorcluster, "Opt_Selector.lvclass"=w3336:refnum<class "Opt_Selector.lvclass">)  [unwired: 7 in, 1 out]
            n1502 = call-dynamic "Read sequencia.vi"("error in (no error)"=w3334, "Opt_Selector in"=w3336) -> ("error out"=w3330:errorcluster, "sequencia"=w3329:u16)  [unwired: 7 in, 1 out]
            n1503 = case shown="True" w3348 {
              tunnel: [0 w3360] -> w3338
              tunnel: w3329 -> [_ w3359]
              frame False {
                # "OV 20230424: \n#SEQ agora armazena as\nposições da lâmina utilizadas.\nNa fotometria, #SEQ=0"
                # "fotometria:"
              }
              frame True {
                # "polarimetria:"
                n1504 = disable-structure shown="Enabled" {
                  disable-tunnel: [w3361 w3363] -> w3360
                  disable-tunnel: w3359 -> [_ w3364]
                  frame Disabled {
                    n1505 = property on="#Polarimetric Sequence Done" class="Slide (strict)"() -> ("Scale.Maximum"=w3362:dbl)  [unwired: 2 in, 2 out]
                    n1506 = To Unsigned Long Integer(number=w3362) -> (unsigned 32bit integer=w3361:u32)
                  }
                  frame Enabled {
                    # "OV 20230424: \n#SEQ agora armazena as\nposições da lâmina utilizadas.\nNa polarimetria, #SEQ=WPROT.sequencia"
                    n1507 = To Unsigned Long Integer(number=w3364) -> (unsigned 32bit integer=w3363:u32)
                  }
                }
              }
            }
            n1508 = call-dynamic "Write Obs_state.vi"("error in (no error)"=w3330, "Obs_state"=u32 251, "S4ACS_GUI in"=w3332) -> ("error out"=w3356:errorcluster, "S4ACS_GUI out"=w3355:refnum<class "S4GUI.lvclass">)  [unwired: 7 in]
            n1509 = local read "# Cycles"() -> (w3343:u32)
            n1510 = stacked-sequence {
              seq-local: [w3386 _ _ _] -> [_ w3465 _ _]
              seq-local: [w3385 _ _ _] -> [_ w3464 _ _]
              seq-local: [_ w3463 _ _] -> [_ _ w3517 _]
              seq-local: [_ w3462 _ _] -> [_ _ w3516 _]
              seq-local: [_ _ w3515 _] -> [_ _ _ w3569]
              seq-local: [_ _ w3514 _] -> [_ _ _ w3568]
              tunnel: w3356 -> [w3406 _ _ _]
              tunnel: w3355 -> [w3405 _ _ _]
              tunnel: [_ _ _ w3567] -> w3340
              tunnel: [_ _ _ w3566] -> w3342
              tunnel: w3353 -> [w3382 w3461 w3513 w3565]
              tunnel: w3352 -> [w3380 w3460 w3481 w3533]
              tunnel: w3351 -> [w3379 w3428 w3480 w3532]
              tunnel: w3350 -> [w3378 w3427 w3479 w3531]
              tunnel: w3349 -> [w3373 w3422 w3474 w3526]
              tunnel: w3343 -> [w3370 w3419 w3471 w3523]
              tunnel: w3338 -> [w3365 w3414 w3466 w3518]
              frame #0 {
                # "object"
                # "suffix"
                # "obsType"
                n1511 = local read "Exptime ch1"() -> (w3381:dbl)
                n1512 = call-dynamic "Read AcquisitionA.vi"("error in (no error)"=w3406, "S4ACS_GUI in"=w3405) -> ("error out"=w3404:errorcluster, "Acquisition.lvclass"=w3403:refnum<class "Acquisition.lvclass">, "S4ACS_GUI out"=w3393:refnum<class "S4GUI.lvclass">)  [unwired: 7 in]
                n1513 = call-dynamic "Read Channel.vi"("error in (no error)"=w3404, "Acquisition in"=w3403) -> ("error out"=w3401:errorcluster, "Channel.lvclass"=w3402:refnum<class "Channel.lvclass">, "Acquisition out"=w3392:refnum<class "Acquisition.lvclass">)  [unwired: 7 in]
                n1514 = local read "Exp ch1"() -> (w3388:u32)
                n1515 = call-dynamic "Read Interface.vi"("error in (no error)"=w3401, "Channel in"=w3402) -> ("error out"=w3413:errorcluster, "Interface.lvclass"=w3399:refnum<class "Interface.lvclass">, "Channel out"=w3400:refnum<class "Channel.lvclass">)  [unwired: 7 in]
                n1516 = call "Write Exposure Time.vi"("error in (no error)"=w3413, "Exposure Time"=w3381, "Interface in"=w3399) -> ("error out"=w3384:errorcluster, "Interface out"=w3383:refnum<class "Interface.lvclass">)  [unwired: 7 in]
                n1517 = call-dynamic "Write Suffix.vi"("error in (no error)"=w3384, "Suffix"=w3382, "Interface in"=w3383) -> ("error out"=w3412:errorcluster, "Interface out"=w3398:refnum<class "Interface.lvclass">)  [unwired: 7 in]
                n1518 = call-dynamic "Write ObsType.vi"("error in (no error)"=w3412, "ObsType"=w3379, "Interface in"=w3398) -> ("error out"=w3411:errorcluster, "Interface out"=w3397:refnum<class "Interface.lvclass">)  [unwired: 7 in]
                n1519 = call-dynamic "Write Object.vi"("error in (no error)"=w3411, "Object"=w3378, "Interface in"=w3397) -> ("error out"=w3410:errorcluster, "Interface out"=w3396:refnum<class "Interface.lvclass">)  [unwired: 7 in]
                n1520 = call-dynamic "Write Comments.vi"("error in (no error)"=w3410, "Comments"=w3380, "Interface in"=w3396) -> ("error out"=w3409:errorcluster, "Interface out"=w3395:refnum<class "Interface.lvclass">)  [unwired: 7 in]
                n1521 = call-dynamic "Write DS9.vi"("error in (no error)"=w3409, "DS9"="F", "Interface in"=w3395) -> ("error out"=w3375:errorcluster, "Interface out"=w3377:refnum<class "Interface.lvclass">)  [unwired: 7 in]
                n1522 = call-dynamic "Write Observer.vi"("error in (no error)"=w3375, "Observer"=w3373, "Interface in"=w3377) -> ("error out"=w3374:errorcluster, "Interface out"=w3376:refnum<class "Interface.lvclass">)  [unwired: 7 in]
                n1523 = call-dynamic "Write # Images.vi"("error in (no error)"=w3374, "# Images"=w3388, "Interface in"=w3376) -> ("error out"=w3407:errorcluster, "Interface out"=w3394:refnum<class "Interface.lvclass">)  [unwired: 7 in]
                n1524 = property on="Exposure Done ch1" class="Slide (strict)"("Scale.Maximum"=w3388, "Scale.Minimum"=0.0 ("Scale.Range:Minimum")) -> ()  [unwired: 2 in, 2 out]
                n1525 = property on="Exposure Time ch1" class="Slide (strict)"("Scale.Maximum"=w3381, "Scale.Minimum"=0.0 ("Scale.Range:Minimum")) -> ()  [unwired: 2 in, 2 out]
                n1526 = call-dynamic "Write Interface.vi"("error in (no error)"=w3407, "Interface.lvclass"=w3394, "Channel in"=w3400) -> ("error out"=w3372:errorcluster, "Channel out"=w3371:refnum<class "Channel.lvclass">)  [unwired: 7 in]
                n1527 = call-dynamic "Write ciclos.vi"("error in (no error)"=w3372, "ciclos"=w3370, "Channel in"=w3371) -> ("error out"=w3367:errorcluster, "Channel out"=w3369:refnum<class "Channel.lvclass">)  [unwired: 7 in]
                n1528 = call-dynamic "Write sequencias.vi"("error in (no error)"=w3367, "sequencias"=w3365, "Channel in"=w3369) -> ("error out"=w3366:errorcluster, "Channel out"=w3368:refnum<class "Channel.lvclass">)  [unwired: 7 in]
                n1529 = call-dynamic "Write Channel.vi"("error in (no error)"=w3366, "Channel.lvclass"=w3368, "Acquisition in"=w3392) -> ("error out"=w3390:errorcluster, "Acquisition out"=w3391:refnum<class "Acquisition.lvclass">)  [unwired: 7 in]
                n1530 = call-dynamic "Write AcquisitionA.vi"("error in (no error)"=w3390, "Acquisition.lvclass"=w3391, "S4ACS_GUI in"=w3393) -> ("error out"=w3385:errorcluster, "S4ACS_GUI out"=w3386:refnum<class "S4GUI.lvclass">)  [unwired: 7 in]
              }
              frame #1 {
                # "object"
                # "suffix"
                # "obsType"
                n1531 = call "Read AcquisitionB.vi"("error in (no error)"=w3464, "S4ACS_GUI in"=w3465) -> ("error out"=w3443:errorcluster, "Acquisition.lvclass"=w3444:refnum<class "Acquisition.lvclass">, "S4ACS_GUI out"=w3456:refnum<class "S4GUI.lvclass">)  [unwired: 7 in]
                n1532 = local read "Exptime ch2"() -> (w3429:dbl)
                n1533 = call-dynamic "Read Channel.vi"("error in (no error)"=w3443, "Acquisition in"=w3444) -> ("error out"=w3446:errorcluster, "Channel.lvclass"=w3445:refnum<class "Channel.lvclass">, "Acquisition out"=w3457:refnum<class "Acquisition.lvclass">)  [unwired: 7 in]
                n1534 = call-dynamic "Read Interface.vi"("error in (no error)"=w3446, "Channel in"=w3445) -> ("error out"=w3435:errorcluster, "Interface.lvclass"=w3448:refnum<class "Interface.lvclass">, "Channel out"=w3447:refnum<class "Channel.lvclass">)  [unwired: 7 in]
                n1535 = call "Write Exposure Time.vi"("error in (no error)"=w3435, "Exposure Time"=w3429, "Interface in"=w3448) -> ("error out"=w3436:errorcluster, "Interface out"=w3449:refnum<class "Interface.lvclass">)  [unwired: 7 in]
                n1536 = call-dynamic "Write # Index.vi"("error in (no error)"=w3436, "# Index"=u32 1, "Interface in"=w3449) -> ("error out"=w3437:errorcluster, "Interface out"=w3450:refnum<class "Interface.lvclass">)  [unwired: 7 in]
                n1537 = call-dynamic "Write Suffix.vi"("error in (no error)"=w3437, "Suffix"=w3461, "Interface in"=w3450) -> ("error out"=w3438:errorcluster, "Interface out"=w3451:refnum<class "Interface.lvclass">)  [unwired: 7 in]
                n1538 = call-dynamic "Write ObsType.vi"("error in (no error)"=w3438, "ObsType"=w3428, "Interface in"=w3451) -> ("error out"=w3439:errorcluster, "Interface out"=w3452:refnum<class "Interface.lvclass">)  [unwired: 7 in]
                n1539 = call-dynamic "Write Object.vi"("error in (no error)"=w3439, "Object"=w3427, "Interface in"=w3452) -> ("error out"=w3440:errorcluster, "Interface out"=w3453:refnum<class "Interface.lvclass">)  [unwired: 7 in]
                n1540 = call-dynamic "Write Comments.vi"("error in (no error)"=w3440, "Comments"=w3460, "Interface in"=w3453) -> ("error out"=w3441:errorcluster, "Interface out"=w3454:refnum<class "Interface.lvclass">)  [unwired: 7 in]
                n1541 = local read "Exp ch2"() -> (w3432:u32)
                n1542 = call-dynamic "Write DS9.vi"("error in (no error)"=w3441, "DS9"="F", "Interface in"=w3454) -> ("error out"=w3424:errorcluster, "Interface out"=w3426:refnum<class "Interface.lvclass">)  [unwired: 7 in]
                n1543 = call-dynamic "Write Observer.vi"("error in (no error)"=w3424, "Observer"=w3422, "Interface in"=w3426) -> ("error out"=w3423:errorcluster, "Interface out"=w3425:refnum<class "Interface.lvclass">)  [unwired: 7 in]
                n1544 = call-dynamic "Write # Images.vi"("error in (no error)"=w3423, "# Images"=w3432, "Interface in"=w3425) -> ("error out"=w3442:errorcluster, "Interface out"=w3455:refnum<class "Interface.lvclass">)  [unwired: 7 in]
                n1545 = property on="Exposure Time ch2" class="Slide (strict)"("Scale.Maximum"=w3429, "Scale.Minimum"=0.0 ("Scale.Range:Minimum")) -> ()  [unwired: 2 in, 2 out]
                n1546 = property on="Exposure Done ch2" class="Slide (strict)"("Scale.Maximum"=w3432, "Scale.Minimum"=0.0 ("Scale.Range:Minimum")) -> ()  [unwired: 2 in, 2 out]
                n1547 = call-dynamic "Write Interface.vi"("error in (no error)"=w3442, "Interface.lvclass"=w3455, "Channel in"=w3447) -> ("error out"=w3421:errorcluster, "Channel out"=w3420:refnum<class "Channel.lvclass">)  [unwired: 7 in]
                n1548 = call-dynamic "Write ciclos.vi"("error in (no error)"=w3421, "ciclos"=w3419, "Channel in"=w3420) -> ("error out"=w3416:errorcluster, "Channel out"=w3418:refnum<class "Channel.lvclass">)  [unwired: 7 in]
                n1549 = call-dynamic "Write sequencias.vi"("error in (no error)"=w3416, "sequencias"=w3414, "Channel in"=w3418) -> ("error out"=w3415:errorcluster, "Channel out"=w3417:refnum<class "Channel.lvclass">)  [unwired: 7 in]
                n1550 = call-dynamic "Write Channel.vi"("error in (no error)"=w3415, "Channel.lvclass"=w3417, "Acquisition in"=w3457) -> ("error out"=w3459:errorcluster, "Acquisition out"=w3458:refnum<class "Acquisition.lvclass">)  [unwired: 7 in]
                n1551 = call "Write AcquisitionB.vi"("error in (no error)"=w3459, "Acquisition.lvclass"=w3458, "S4ACS_GUI in"=w3456) -> ("error out"=w3462:errorcluster, "S4ACS_GUI out"=w3463:refnum<class "S4GUI.lvclass">)  [unwired: 7 in]
              }
              frame #2 {
                # "object"
                # "suffix"
                # "obsType"
                n1552 = call-dynamic "Read AcquisitionC.vi"("error in (no error)"=w3516, "S4ACS_GUI in"=w3517) -> ("error out"=w3504:errorcluster, "Acquisition.lvclass"=w3503:refnum<class "Acquisition.lvclass">, "S4ACS_GUI out"=w3491:refnum<class "S4GUI.lvclass">)  [unwired: 7 in]
                n1553 = call-dynamic "Read Channel.vi"("error in (no error)"=w3504, "Acquisition in"=w3503) -> ("error out"=w3501:errorcluster, "Channel.lvclass"=w3502:refnum<class "Channel.lvclass">, "Acquisition out"=w3490:refnum<class "Acquisition.lvclass">)  [unwired: 7 in]
                n1554 = local read "Exptime ch3"() -> (w3487:dbl)
                n1555 = call-dynamic "Read Interface.vi"("error in (no error)"=w3501, "Channel in"=w3502) -> ("error out"=w3512:errorcluster, "Interface.lvclass"=w3499:refnum<class "Interface.lvclass">, "Channel out"=w3500:refnum<class "Channel.lvclass">)  [unwired: 7 in]
                n1556 = call "Write Exposure Time.vi"("error in (no error)"=w3512, "Exposure Time"=w3487, "Interface in"=w3499) -> ("error out"=w3511:errorcluster, "Interface out"=w3498:refnum<class "Interface.lvclass">)  [unwired: 7 in]
                n1557 = call-dynamic "Write # Index.vi"("error in (no error)"=w3511, "# Index"=u32 1, "Interface in"=w3498) -> ("error out"=w3510:errorcluster, "Interface out"=w3497:refnum<class "Interface.lvclass">)  [unwired: 7 in]
                n1558 = call-dynamic "Write Suffix.vi"("error in (no error)"=w3510, "Suffix"=w3513, "Interface in"=w3497) -> ("error out"=w3509:errorcluster, "Interface out"=w3496:refnum<class "Interface.lvclass">)  [unwired: 7 in]
                n1559 = call-dynamic "Write ObsType.vi"("error in (no error)"=w3509, "ObsType"=w3480, "Interface in"=w3496) -> ("error out"=w3508:errorcluster, "Interface out"=w3495:refnum<class "Interface.lvclass">)  [unwired: 7 in]
                n1560 = call-dynamic "Write Object.vi"("error in (no error)"=w3508, "Object"=w3479, "Interface in"=w3495) -> ("error out"=w3507:errorcluster, "Interface out"=w3494:refnum<class "Interface.lvclass">)  [unwired: 7 in]
                n1561 = call-dynamic "Write Comments.vi"("error in (no error)"=w3507, "Comments"=w3481, "Interface in"=w3494) -> ("error out"=w3506:errorcluster, "Interface out"=w3493:refnum<class "Interface.lvclass">)  [unwired: 7 in]
                n1562 = call-dynamic "Write DS9.vi"("error in (no error)"=w3506, "DS9"="F", "Interface in"=w3493) -> ("error out"=w3476:errorcluster, "Interface out"=w3478:refnum<class "Interface.lvclass">)  [unwired: 7 in]
                n1563 = local read "Exp ch3"() -> (w3484:u32)
                n1564 = property on="Exposure Time ch3" class="Slide (strict)"("Scale.Maximum"=w3487, "Scale.Minimum"=0.0 ("Scale.Range:Minimum")) -> ()  [unwired: 2 in, 2 out]
                n1565 = call-dynamic "Write Observer.vi"("error in (no error)"=w3476, "Observer"=w3474, "Interface in"=w3478) -> ("error out"=w3475:errorcluster, "Interface out"=w3477:refnum<class "Interface.lvclass">)  [unwired: 7 in]
                n1566 = property on="Exposure Done ch3" class="Slide (strict)"("Scale.Maximum"=w3484, "Scale.Minimum"=0.0 ("Scale.Range:Minimum")) -> ()  [unwired: 2 in, 2 out]
                n1567 = call-dynamic "Write # Images.vi"("error in (no error)"=w3475, "# Images"=w3484, "Interface in"=w3477) -> ("error out"=w3505:errorcluster, "Interface out"=w3492:refnum<class "Interface.lvclass">)  [unwired: 7 in]
                n1568 = call-dynamic "Write Interface.vi"("error in (no error)"=w3505, "Interface.lvclass"=w3492, "Channel in"=w3500) -> ("error out"=w3473:errorcluster, "Channel out"=w3472:refnum<class "Channel.lvclass">)  [unwired: 7 in]
                n1569 = call-dynamic "Write ciclos.vi"("error in (no error)"=w3473, "ciclos"=w3471, "Channel in"=w3472) -> ("error out"=w3468:errorcluster, "Channel out"=w3470:refnum<class "Channel.lvclass">)  [unwired: 7 in]
                n1570 = call-dynamic "Write sequencias.vi"("error in (no error)"=w3468, "sequencias"=w3466, "Channel in"=w3470) -> ("error out"=w3467:errorcluster, "Channel out"=w3469:refnum<class "Channel.lvclass">)  [unwired: 7 in]
                n1571 = call-dynamic "Write Channel.vi"("error in (no error)"=w3467, "Channel.lvclass"=w3469, "Acquisition in"=w3490) -> ("error out"=w3488:errorcluster, "Acquisition out"=w3489:refnum<class "Acquisition.lvclass">)  [unwired: 7 in]
                n1572 = call-dynamic "Write AcquisitionC.vi"("error in (no error)"=w3488, "Acquisition.lvclass"=w3489, "S4ACS_GUI in"=w3491) -> ("error out"=w3514:errorcluster, "S4ACS_GUI out"=w3515:refnum<class "S4GUI.lvclass">)  [unwired: 7 in]
              }
              frame #3 {
                # "object"
                # "suffix"
                # "obsType"
                n1573 = call-dynamic "Read AcquisitionD.vi"("error in (no error)"=w3568, "S4ACS_GUI in"=w3569) -> ("error out"=w3556:errorcluster, "Acquisition.lvclass"=w3555:refnum<class "Acquisition.lvclass">, "S4ACS_GUI out"=w3543:refnum<class "S4GUI.lvclass">)  [unwired: 7 in]
                n1574 = call-dynamic "Read Channel.vi"("error in (no error)"=w3556, "Acquisition in"=w3555) -> ("error out"=w3553:errorcluster, "Channel.lvclass"=w3554:refnum<class "Channel.lvclass">, "Acquisition out"=w3542:refnum<class "Acquisition.lvclass">)  [unwired: 7 in]
                n1575 = local read "Exptime ch4"() -> (w3538:dbl)
                n1576 = call-dynamic "Read Interface.vi"("error in (no error)"=w3553, "Channel in"=w3554) -> ("error out"=w3564:errorcluster, "Interface.lvclass"=w3551:refnum<class "Interface.lvclass">, "Channel out"=w3552:refnum<class "Channel.lvclass">)  [unwired: 7 in]
                n1577 = call "Write Exposure Time.vi"("error in (no error)"=w3564, "Exposure Time"=w3538, "Interface in"=w3551) -> ("error out"=w3563:errorcluster, "Interface out"=w3550:refnum<class "Interface.lvclass">)  [unwired: 7 in]
                n1578 = call-dynamic "Write # Index.vi"("error in (no error)"=w3563, "# Index"=u32 1, "Interface in"=w3550) -> ("error out"=w3562:errorcluster, "Interface out"=w3549:refnum<class "Interface.lvclass">)  [unwired: 7 in]
                n1579 = call-dynamic "Write Suffix.vi"("error in (no error)"=w3562, "Suffix"=w3565, "Interface in"=w3549) -> ("error out"=w3561:errorcluster, "Interface out"=w3548:refnum<class "Interface.lvclass">)  [unwired: 7 in]
                n1580 = call-dynamic "Write ObsType.vi"("error in (no error)"=w3561, "ObsType"=w3532, "Interface in"=w3548) -> ("error out"=w3560:errorcluster, "Interface out"=w3547:refnum<class "Interface.lvclass">)  [unwired: 7 in]
                n1581 = call-dynamic "Write Object.vi"("error in (no error)"=w3560, "Object"=w3531, "Interface in"=w3547) -> ("error out"=w3559:errorcluster, "Interface out"=w3546:refnum<class "Interface.lvclass">)  [unwired: 7 in]
                n1582 = call-dynamic "Write Comments.vi"("error in (no error)"=w3559, "Comments"=w3533, "Interface in"=w3546) -> ("error out"=w3558:errorcluster, "Interface out"=w3545:refnum<class "Interface.lvclass">)  [unwired: 7 in]
                n1583 = call-dynamic "Write DS9.vi"("error in (no error)"=w3558, "DS9"="F", "Interface in"=w3545) -> ("error out"=w3528:errorcluster, "Interface out"=w3530:refnum<class "Interface.lvclass">)  [unwired: 7 in]
                n1584 = property on="Exposure Time ch4" class="Slide (strict)"("Scale.Maximum"=w3538, "Scale.Minimum"=0.0 ("Scale.Range:Minimum")) -> ()  [unwired: 2 in, 2 out]
                n1585 = local read "Exp ch4"() -> (w3536:u32)
                n1586 = call-dynamic "Write Observer.vi"("error in (no error)"=w3528, "Observer"=w3526, "Interface in"=w3530) -> ("error out"=w3527:errorcluster, "Interface out"=w3529:refnum<class "Interface.lvclass">)  [unwired: 7 in]
                n1587 = property on="Exposure Done ch4" class="Slide (strict)"("Scale.Maximum"=w3536, "Scale.Minimum"=0.0 ("Scale.Range:Minimum")) -> ()  [unwired: 2 in, 2 out]
                n1588 = call-dynamic "Write # Images.vi"("error in (no error)"=w3527, "# Images"=w3536, "Interface in"=w3529) -> ("error out"=w3557:errorcluster, "Interface out"=w3544:refnum<class "Interface.lvclass">)  [unwired: 7 in]
